vi "End.vi"(8 "error in (no error)":errorcluster, 11 "Simulated_CCD_Camera in":refnum<class "Simulated Camera.lvclass">) -> (0 "error out":errorcluster, 3 "Simulated_CCD_Camera out":refnum<class "Simulated Camera.lvclass">)   [LabVIEW 2018, in "Simulated Camera.lvclass"]
doc: "Correctly ends communication with the camera."
uses:
  Simulated Camera.lvclass
  Simulated Camera.lvclass/Simulated Camera.ctl
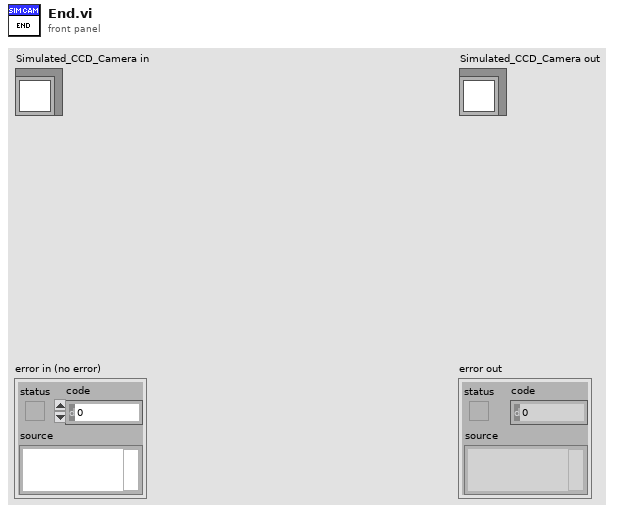
[diagram p1: front panel]
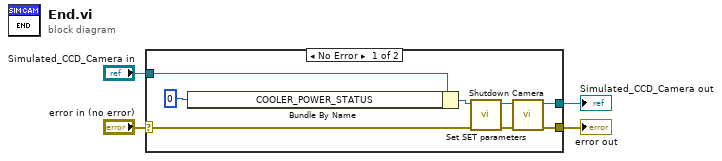
[diagram p0: block diagram]
diagram:
  n1 = case shown="No Error" "error in (no error)" {
    selector: "error in (no error)" -> [w9 w14]
    tunnel: [w8 w14] -> w3
    tunnel: [w7 w13] -> w1
    tunnel: "Simulated_CCD_Camera in" -> [w6 w13]
    frame No Error {
      n2 = Bundle By Name(cluster=w6, "COOLER_POWER_STATUS"=u16 0) -> (w5:refnum<class "Simulated Camera.lvclass">)
      n3 = call-dynamic "Set SET parameters.vi"("error in (no error)"=w9, "Simulated_CCD_Camera in"=w5) -> ("error out"=w10:errorcluster, "Simulated_CCD_Camera out"=w11:refnum<class "Simulated Camera.lvclass">)  [unwired: 8 in]
      n4 = call-dynamic "Shutdown Camera.vi"("error in (no error)"=w10, "CCDCamera in"=w11) -> ("error out"=w8:errorcluster, "CCDCamera out"=w7:refnum<class "Simulated Camera.lvclass">)  [unwired: 8 in]
    }
    frame Error {
    }
  }
  "error out" <- w3
  "Simulated_CCD_Camera out" <- w1
